vi "obj_DataLog Current Database Info.vi"(0 "method":T8, 1 "initial number (NaN)":dbl=nan format="%.2f", 5 "tag or base tag":string, 7 "tag config in":T3 {"logging parameters" format="%.2e"; "precision" items=["0", "1", "2", "3", "4", "5", "6", "7", "8", "9", "10", "11", "12", "13", "14", "15", "16", "17"]; "limit delay" format="%.2e"; "deadband" format="%.2e"}, 9 "tag index/change#":i32, 11 "error in (no error)":errorcluster, 12 "meta specifier (not a meta)":T2=enum."not a meta", 13 "initial string (\"\")":string) -> (3 "mode":T1, 4 "tag config list":T3[](array[typedef]) {"logging parameters" format="%.2e"; "precision" items=["0", "1", "2", "3", "4", "5", "6", "7", "8", "9", "10", "11", "12", "13", "14", "15", "16", "17"]; "limit delay" format="%.2e"; "deadband" format="%.2e"}, 6 "#tags/change#":i32, 8 "tag config out":T3 {"logging parameters" format="%.2e"; "precision" items=["0", "1", "2", "3", "4", "5", "6", "7", "8", "9", "10", "11", "12", "13", "14", "15", "16", "17"]; "limit delay" format="%.2e"; "deadband" format="%.2e"}, 10 "dup tag index":i32, 14 "path":path, 15 "error out":errorcluster)   [LabVIEW 2012]
uses:
  typedefs/t_DataLog Tag Info List Methods.ctl
  typedefs/t_Datalog Datebase Modes.ctl
  typedefs/clusters/t_DataLog Tag Config.ctl
  typedefs/t_DataLog Temporal Types.ctl
  typedefs/t_DataLog Value Types.ctl
  typedefs/t_DataLog Numerical Format.ctl
  typedefs/t_DataLog Logging Algorithms.ctl
  typedefs/et_DataLog Meta Tag Specifier.ctl
  typedefs/t_DataLog Databases Methods.ctl
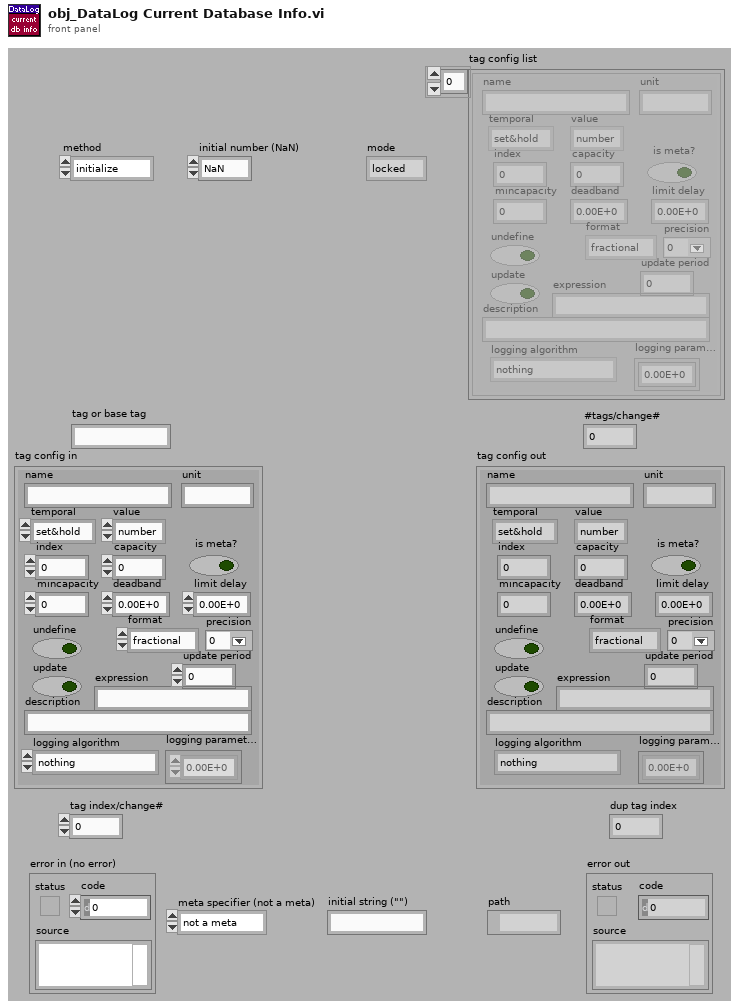
[diagram p1: front panel]
types:
  T1 = typedef "t_Datalog Datebase Modes.ctl" = enum16{"locked", "unlocked", "live", "mirrored"}
  T2 = typedef "et_DataLog Meta Tag Specifier.ctl" = enum32{"warn_lo", "warn_hi", "A_lo", "A_hi", "B_lo", "B_hi", "C_lo", "C_hi", "D_lo", "D_hi", "E_lo", "E_hi", "F_lo", "F_hi", "G_lo", "G_hi", "H_lo", "H_hi", "I_lo", "I_hi", "J_lo", "J_hi", "K_lo", "K_hi", "L_lo", "L_hi", "M_lo", "M_hi", "N_lo", "N_hi", "min", "max", "not a meta"}
  T3 = typedef "t_DataLog Tag Config.ctl" = cluster{"name":string, "unit":string, "temporal":T4, "value":T5, "index":i32, "capacity":i32, "is meta?":bool, "mincapacity":i32, "deadband":dbl, "limit delay":dbl, "format":T6, "precision":u8, "undefine":bool, "update":bool, "update period":u16, "expression":string, "description":string, "logging algorithm":T7, "logging parameters":dbl[]}
  T4 = typedef "t_DataLog Temporal Types.ctl" = enum16{"set&hold", "sample", "event"}
  T5 = typedef "t_DataLog Value Types.ctl" = enum16{"number", "string"}
  T6 = typedef "t_DataLog Numerical Format.ctl" = enum8{"fractional", "exponential", "engineering"}
  T7 = typedef "t_DataLog Logging Algorithms.ctl" = enum16{"nothing", "changes", "everything", "every Nth", "time threshold", "value threshold + prior", "t or v threshold", "t or v threshold + prior"}
  T8 = typedef "t_DataLog Tag Info List Methods.ctl" = enum16{"initialize", "create", "create empty", "rename", "delete", "test tag", "get", "get by name", "get default", "get list", "get path", "get subsets", "set subsets", "set config", "set capacity", "#tags", "go live", "set unlocked", "set mirrored"}
  T9 = typedef "t_DataLog Databases Methods.ctl" = enum16{"initialize", "get ref", "get names", "cleanup"}
  T10 = typedef "t_DataLog Database Info Pane.ctl" = refnum<vi>
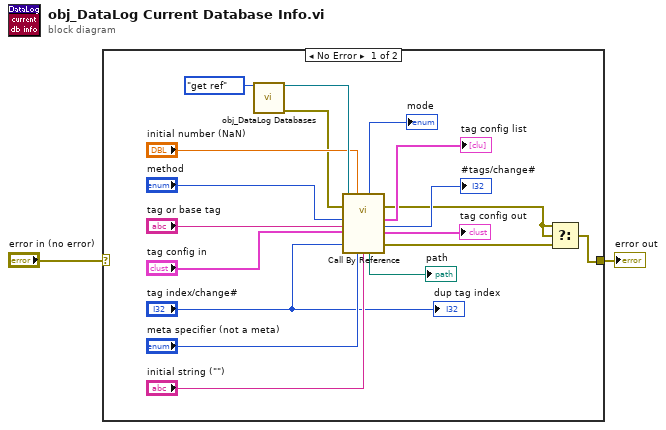
[diagram p0: block diagram]
diagram:
  n1 = case shown="No Error" "error in (no error)" {
    selector: "error in (no error)" -> [_ w21]
    tunnel: [w18 w21] -> w2
    frame No Error {
      n2 = call "obj_DataLog Databases.vi"("method"=t_DataLog_Databases_Methods."get ref") -> ("database ref"=w19:T10, "error out"=w9:errorcluster)  [unwired: 12 in, 1 out]
      n3 = call-by-ref "?"(reference=w19, error in=w9, "method"="method", "initial number (NaN)"="initial number (NaN)", "tag or base tag"="tag or base tag", "tag config in"="tag config in", "tag index/change#"="tag index/change#", "meta specifier (not a meta)"="meta specifier (not a meta)", "initial string (\"\")"="initial string (\"\")") -> (error out=w6:errorcluster, "mode"=→"mode":T1, "tag config list"=→"tag config list":T3[], "#tags/change#"=→"#tags/change#":i32, "tag config out"=→"tag config out":T3, "path"=→"path":path, 15:"error out"=w7:errorcluster)  [unwired: 2 in, 2 out]
      n4 = Select(t=w6, s=w6, f=w7) -> (s? t:f=w18:errorcluster)
      "dup tag index" <- "tag index/change#"
    }
    frame Error {
    }
  }
  "error out" <- w2
